vi "REMOND Studio_EC Water Q.vi"() -> ()   [LabVIEW 2021]
uses:
  FSM_States.ctl
  Global_Message.ctl
  <vilib>/Utility/error.llb/DialogType.ctl
  <vilib>/Modbus/master/Modbus Master.lvclass
  Global_flags.vi
  <vilib>/Modbus/master/Create Master Instance (Serial).vi
panel:
  in  "D.S":u16(ring)=1 items=["0.5s", "1s", "1.5s", "2.0s", "2.5s", "3.0s", "3.5s", "4.0s", "4.5s", "5.0s"]
  out "New EC":sgl=1.0
  in  "Standard Sol [mS/cm].":sgl=1.413
  in  "Set K=1":bool
  in  "Confirm EC":bool
  in  "BaudRate (9600)":u32=9600
  in  "Address":u8=1
  in  "Open/Close COM":bool
  in  "COM":refnum<visa-resource-name>
  out "Salinity:":sgl
  out "TDS:":sgl
  out "Temperature [°C]:":sgl
  out "Resistivity [ohm.cm]:":sgl
  in  "Exit":bool
  in  "Restore Default":bool
  out "Conductivity [mS/cm]:":sgl
  in  "Adquire / Stop":bool
  out "Consumer Shutdown":bool
  in  "SetBaudRate":bool
  in  "BaudRate (9600)":u16(ring)=2 items=["2400", "4800", "9600", "19200", "38400"]
  in  "Addr Set":u16=1
  in  "SetAddress":bool
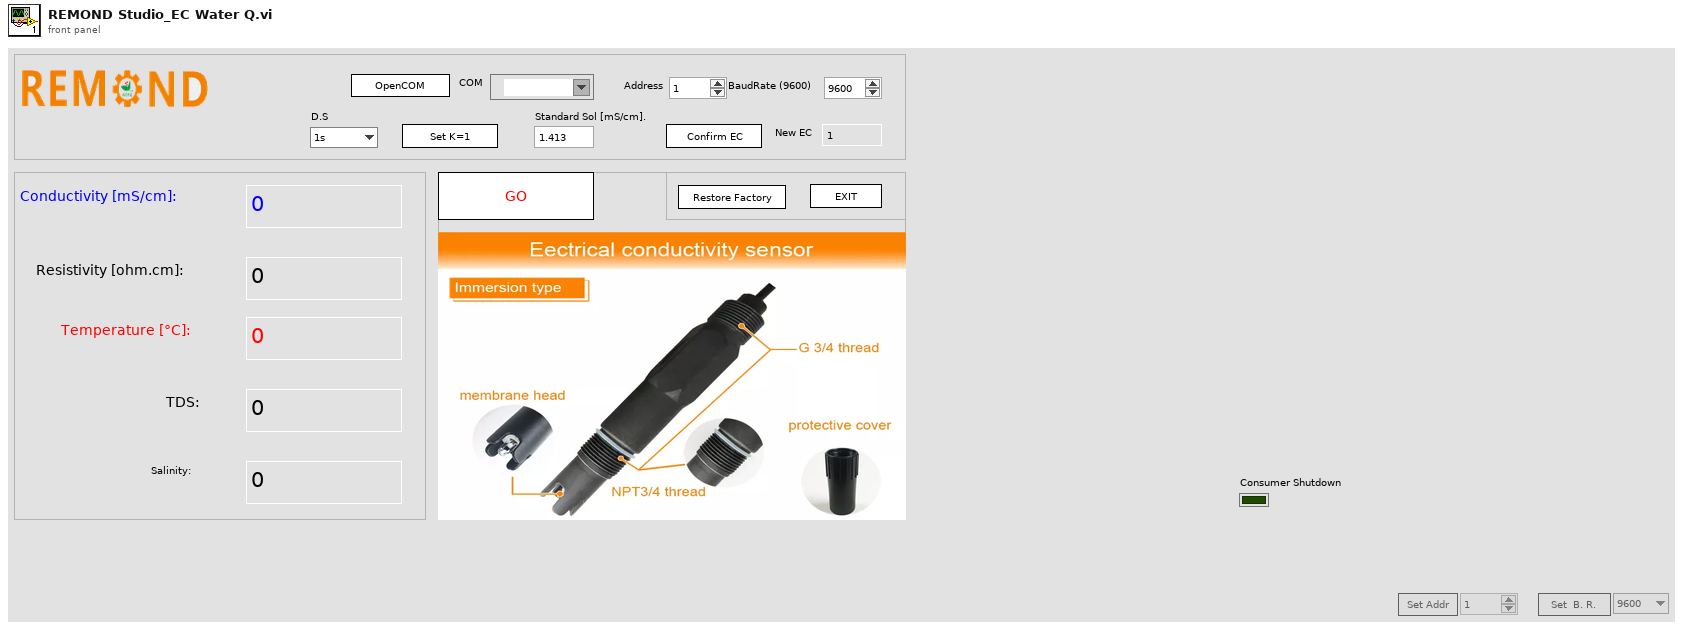
[diagram p1: front panel]
types:
  T1 = typedef "Global_Message.ctl" = cluster{"Consumer State":T2, "User Msg":string, "error in (no error)":errorcluster, "User Msg 2":string}
  T2 = typedef "FSM_States.ctl" = enum16{"Initialize", "Open COM Port", "Adquire Data", "Set Address", "Set BaudRate", "Restore Factory", "Pre-Set Zero", "Pre-Set K=1", "Pre-Set Slope", "Confirm Zero", "Confirm Slope", "Confirm EC", "Close COM Port", "Exit App", "Stop Data", "Calibrate sensor"}
  T3 = typedef "DialogType.ctl" = u16
  T4 = enum8{"Enabled", "Disabled", "Disabled and Grayed Out"}
  T5 = cluster{"Conductivity":sgl, "Resistivity":sgl, "Temperature":sgl, "TDS":sgl, "Salinity":sgl}
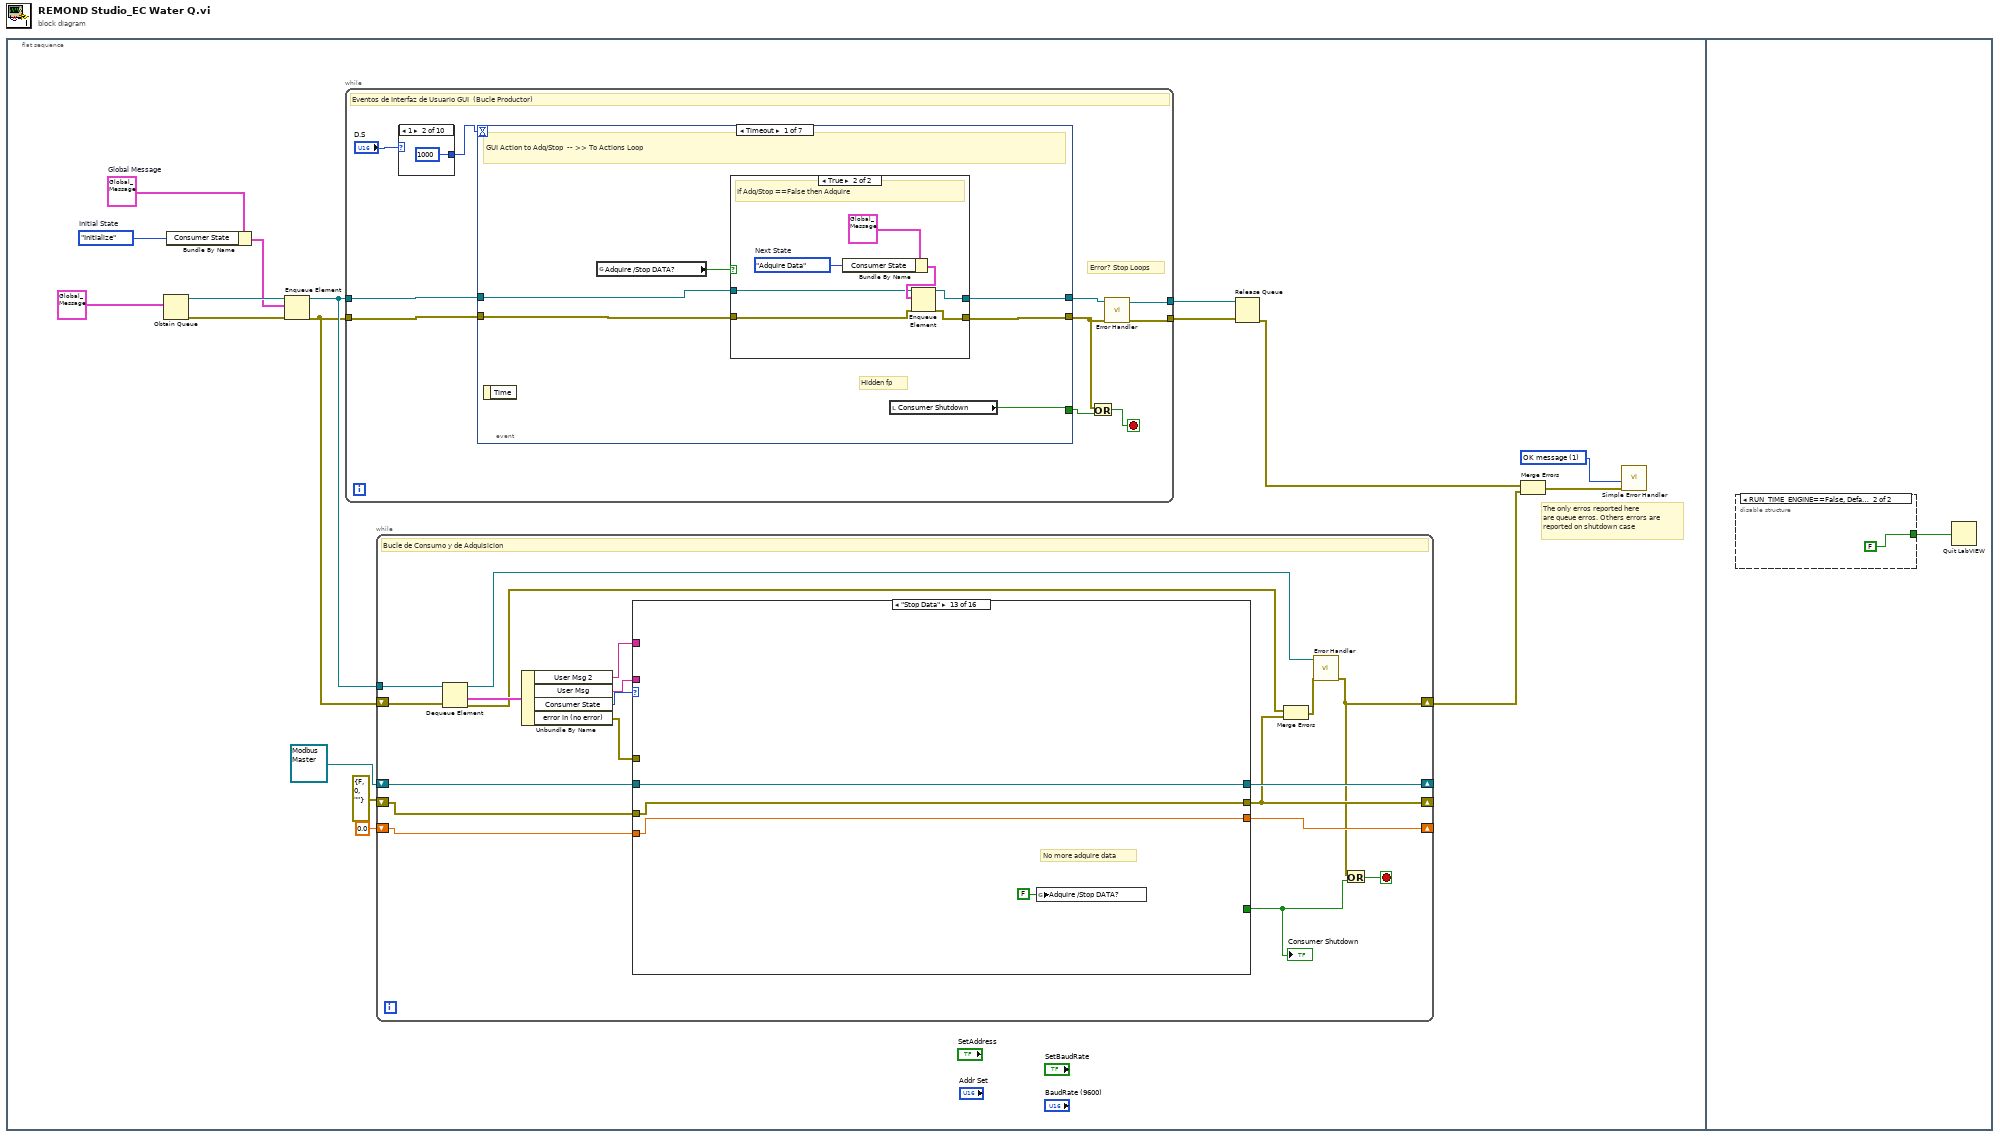
[diagram p0: block diagram]
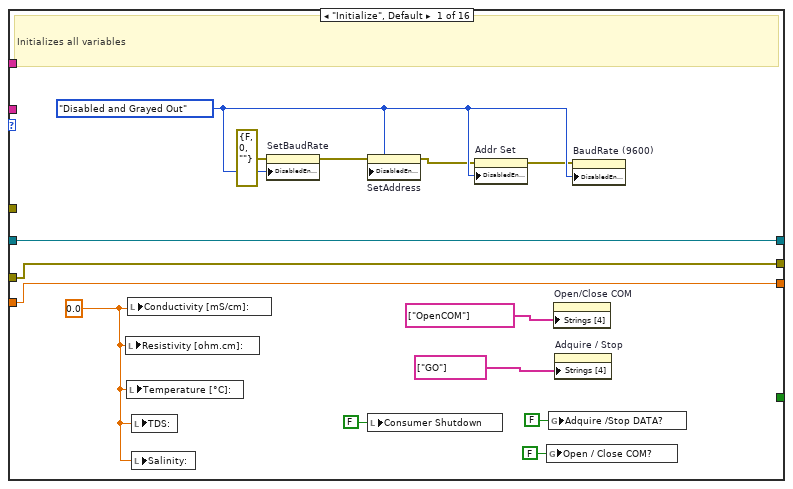
[diagram p2: hidden frame]
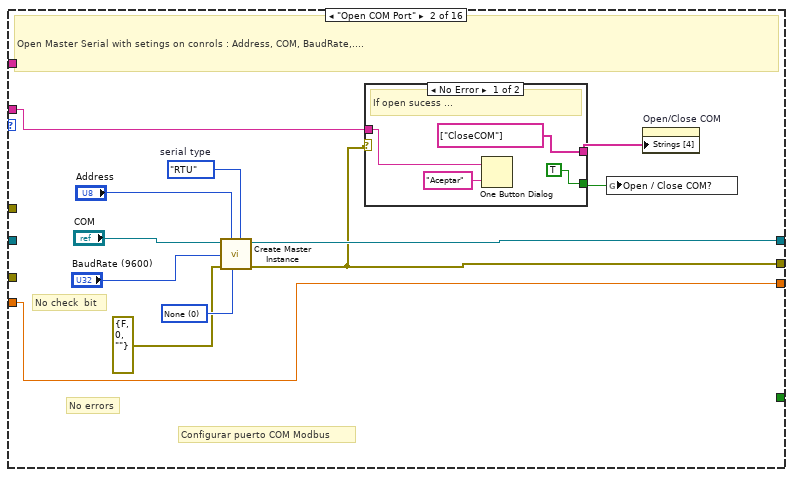
[diagram p3: hidden frame]
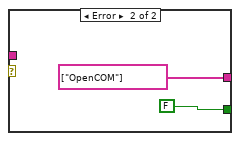
[diagram p4: hidden frame]
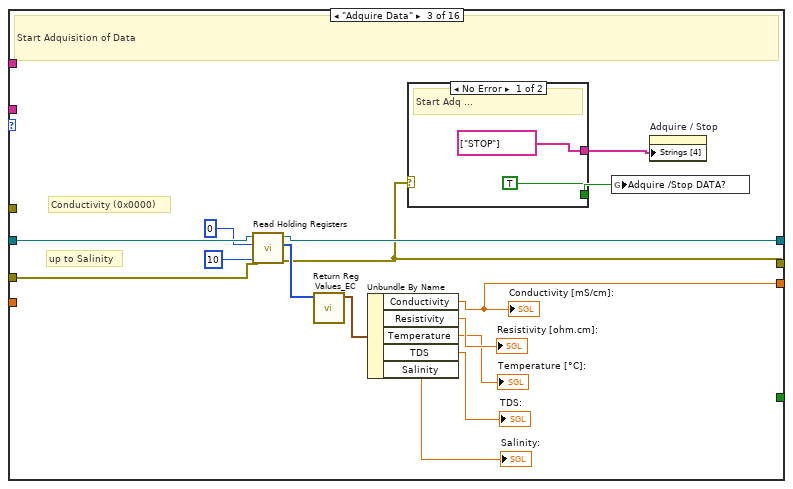
[diagram p5: hidden frame]
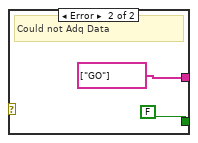
[diagram p6: hidden frame]
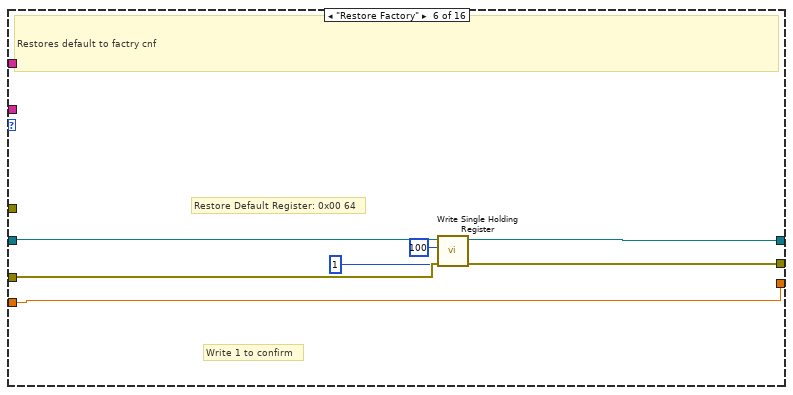
[diagram p9: hidden frame]
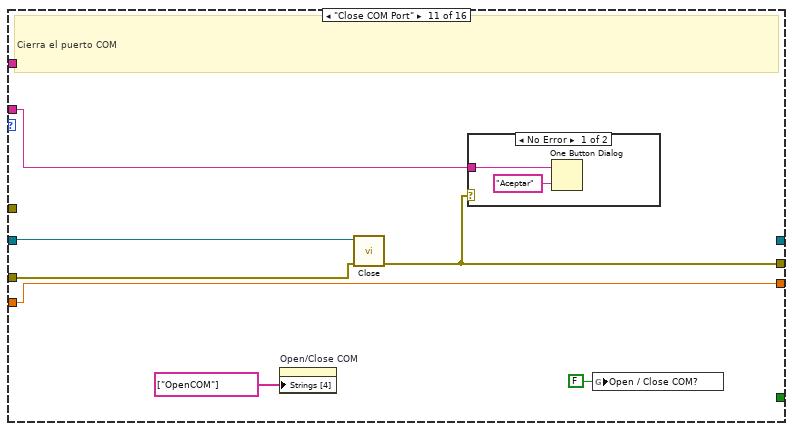
[diagram p14: hidden frame]
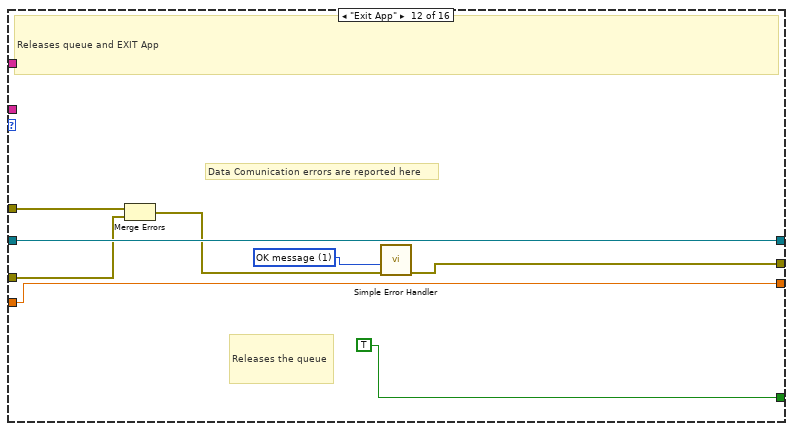
[diagram p16: hidden frame]
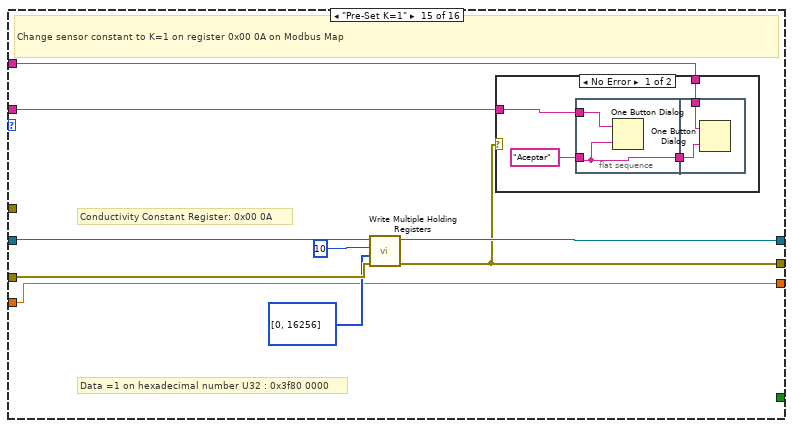
[diagram p18: hidden frame]
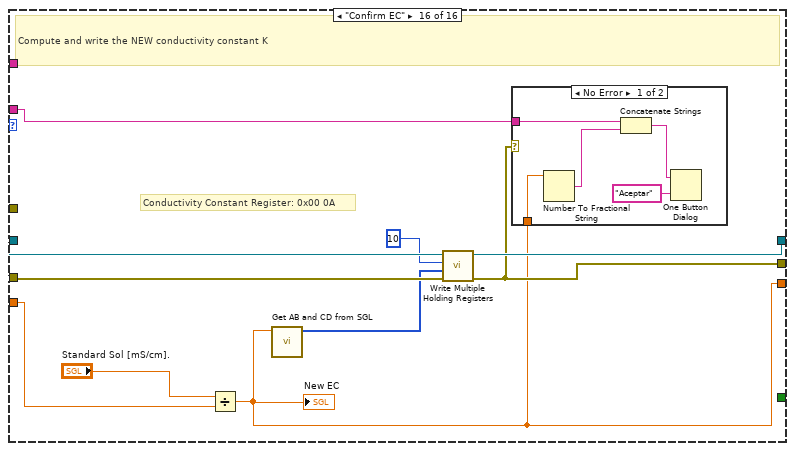
[diagram p20: hidden frame]
diagram:
  n1 = flat-sequence {
    frame #0 {
      w3 = T3 1 items=["no dialog", "OK message", "continue or stop message", "OK message + warnings", "continue/stop + warnings"] ("type of dialog (OK msg:1)")
      w14 = T1 {"Consumer State"=enum."Open COM Port", "User Msg"="", "error in (no error)"={"status"=FALSE, "code"=0, "source"=""}, "User Msg 2"=""}  # Global Message
      w13 = FSM_States."Initialize"  # Initial State
      # "The only erros reported here\nare queue erros. Others errors are\nreported on shutdown case"
      n2 = Obtain Queue(element data type=T1 {"Consumer State"=enum."Open COM Port", "User Msg"="", "error in (no error)"={"status"=FALSE, "code"=0, "source"=""}, "User Msg 2"=""} ("Global Message")) -> (queue out=w16:refnum<queue>, error out=w15:errorcluster)  [unwired: 4 in, 1 out]
      n3 = Bundle By Name(cluster=w14, "Consumer State"=w13) -> (w12:T1)
      n4 = Enqueue Element(queue=w16, element=w12, error in (no error)=w15) -> (queue out=w9:refnum<queue>, error out=w8:errorcluster)  [unwired: 1 in, 1 out]
      n5 = while {
        tunnel: w9 -> [w178]
        tunnel: w8 -> [w177]
        tunnel: [w175] -> w11
        tunnel: [w174] -> w10
        stop <- w173 stop-if-true
        # "Error? Stop Loops"
        # "Eventos de Interfaz de Usuario GUI  (Bucle Productor)"
        n6 = case shown="1" "D.S" {
          tunnel: [500 1000 1500 2000 2500 3000 3500 4000 4500 5000] -> w170
          frame 0, Default {
          }
          frame 1 {
          }
          frame 2 {
          }
          frame 3 {
          }
          frame 4 {
          }
          frame 5 {
          }
          frame 6 {
          }
          frame 7 {
          }
          frame 8 {
          }
          frame 9 {
          }
        }
        n7 = event shown="[0] Timeout" {
          selector: _ -> [_ _ _ _ _ _ _]
          dyn-events: _ -> [_ _ _ _ _ _ _]
          timeout: w170 -> [_ _ _ _ _ _ _]
          tunnel: w178 -> [w194 w208 w221 w242 w249 w256 w265]
          tunnel: w177 -> [w192 w207 w219 w240 w247 w254 w263]
          tunnel: [w193 w205 w220 w241 w248 w255 w264] -> w176
          tunnel: [w191 w204 w218 w239 w246 w253 w262] -> w172
          tunnel: [w189 _ _ _ _ _ TRUE] -> w169
          event Timeout {
            # "Hidden fp"
            # "GUI Action to Adq/Stop  -- >> To Actions Loop"
            n8 = event-data() -> ()  [unwired: 1 in, 1 out]
            n9 = global read "Global_flags.vi" "Adquire /Stop DATA?"() -> (w190:bool)
            n10 = case shown="True" w190 {
              tunnel: w194 -> [w196 w201]
              tunnel: [w196 w200] -> w193
              tunnel: w192 -> [w195 w199]
              tunnel: [w195 w198] -> w191
              frame False {
                # "Otherwise bypass..."
              }
              frame True {
                w197 = FSM_States."Adquire Data"  # Next State
                # "If Adq/Stop ==False then Adquire"
                n11 = Bundle By Name(cluster=T1 {"Consumer State"=enum."Open COM Port", "User Msg"="", "error in (no error)"={"status"=FALSE, "code"=0, "source"=""}, "User Msg 2"=""} ("Global Message"), "Consumer State"=w197) -> (w202:T1)
                n12 = Enqueue Element(queue=w201, element=w202, error in (no error)=w199) -> (queue out=w200:refnum<queue>, error out=w198:errorcluster)  [unwired: 1 in, 1 out]
              }
            }
            n13 = local read "Consumer Shutdown"() -> (w189:bool)
          }
          event "Open/Close COM": Value Change {
            w213 = FSM_States."Close COM Port"  # Next State
            w214 = FSM_States."Open COM Port"  # Next State
            # "GUI Action to Open COM Port  -- >> To Actions Loop"
            n14 = event-data() -> ()  [unwired: 1 in, 1 out]
            n15 = global read "Global_flags.vi" "Open / Close COM?"() -> (w210:bool)
            n16 = Select(t="COM cerrado !", s=w210, f="Puerto COM abierto !" ("User Msg")) -> (s? t:f=w209:string)
            n17 = Select(t=w213, s=w210, f=w214) -> (s? t:f=w216:T2)
            n18 = Bundle By Name(cluster=T1 {"Consumer State"=enum."Open COM Port", "User Msg"="", "error in (no error)"={"status"=FALSE, "code"=0, "source"=""}, "User Msg 2"=""} ("Global Message"), "Consumer State"=w216, "User Msg"=w209) -> (w206:T1)
            n19 = Enqueue Element(queue=w208, element=w206, error in (no error)=w207) -> (queue out=w205:refnum<queue>, error out=w204:errorcluster)  [unwired: 1 in, 1 out]
          }
          event "Adquire / Stop": Value Change {
            # "! Adq has started ?"
            # "GUI Action to Adquire / Stop  -- >> To Actions Loop"
            n20 = event-data() -> ()  [unwired: 1 in, 1 out]
            n21 = global read "Global_flags.vi" "Adquire /Stop DATA?"() -> (w217:bool)
            n22 = case shown="True" w217 {
              tunnel: w221 -> [w226 w232]
              tunnel: [w225 w231] -> w220
              tunnel: w219 -> [w224 w229]
              tunnel: [w223 w230] -> w218
              frame False {
                w222 = FSM_States."Adquire Data"  # Next State
                # "If no Adq started, then Start adquiring .."
                n23 = Bundle By Name(cluster=T1 {"Consumer State"=enum."Open COM Port", "User Msg"="", "error in (no error)"={"status"=FALSE, "code"=0, "source"=""}, "User Msg 2"=""} ("Global Message"), "Consumer State"=w222) -> (w227:T1)
                n24 = Enqueue Element(queue=w226, element=w227, error in (no error)=w224) -> (queue out=w225:refnum<queue>, error out=w223:errorcluster)  [unwired: 1 in, 1 out]
              }
              frame True {
                w233 = FSM_States."Stop Data"  # Next State
                # "Otherwise STOP Adq"
                n25 = Bundle By Name(cluster=T1 {"Consumer State"=enum."Open COM Port", "User Msg"="", "error in (no error)"={"status"=FALSE, "code"=0, "source"=""}, "User Msg 2"=""} ("Global Message"), "Consumer State"=w233) -> (w234:T1)
                n26 = Enqueue Element(queue=w232, element=w234, error in (no error)=w229) -> (queue out=w231:refnum<queue>, error out=w230:errorcluster)  [unwired: 1 in, 1 out]
              }
            }
          }
          event "Set K=1": Value Change {
            w243 = FSM_States."Pre-Set K=1"  # Next State
            # "GUI Action to \"Set K=1\"  -- >> To Actions Loop"
            n27 = event-data() -> ()  [unwired: 1 in, 1 out]
            n28 = Bundle By Name(cluster=T1 {"Consumer State"=enum."Open COM Port", "User Msg"="", "error in (no error)"={"status"=FALSE, "code"=0, "source"=""}, "User Msg 2"=""} ("Global Message"), "Consumer State"=w243, "User Msg"="OK Set K=1 !! ", "User Msg 2"="Colocar sensor en Liqu de calibracion. " ("User Msg")) -> (w238:T1)
            n29 = Enqueue Element(queue=w242, element=w238, error in (no error)=w240) -> (queue out=w241:refnum<queue>, error out=w239:errorcluster)  [unwired: 1 in, 1 out]
          }
          event "Confirm EC": Value Change {
            w252 = FSM_States."Confirm EC"  # Next State
            # "GUI Action to Confirm EC  -- >> To Actions Loop"
            n30 = event-data() -> ()  [unwired: 1 in, 1 out]
            n31 = Bundle By Name(cluster=T1 {"Consumer State"=enum."Open COM Port", "User Msg"="", "error in (no error)"={"status"=FALSE, "code"=0, "source"=""}, "User Msg 2"=""} ("Global Message"), "Consumer State"=w252, "User Msg"="OK Set K=") -> (w250:T1)
            n32 = Enqueue Element(queue=w249, element=w250, error in (no error)=w247) -> (queue out=w248:refnum<queue>, error out=w246:errorcluster)  [unwired: 1 in, 1 out]
          }
          event "Restore Default": Value Change {
            w260 = FSM_States."Restore Factory"  # Next State
            # "GUI Action to Restore Default  -- >> To Actions Loop"
            n33 = event-data() -> ()  [unwired: 1 in, 1 out]
            n34 = Bundle By Name(cluster=T1 {"Consumer State"=enum."Open COM Port", "User Msg"="", "error in (no error)"={"status"=FALSE, "code"=0, "source"=""}, "User Msg 2"=""} ("Global Message"), "Consumer State"=w260, "User Msg"="OK Restore Fact !") -> (w258:T1)
            n35 = Enqueue Element(queue=w256, element=w258, error in (no error)=w254) -> (queue out=w255:refnum<queue>, error out=w253:errorcluster)  [unwired: 1 in, 1 out]
          }
          event "Exit": Value Change {
            w267 = FSM_States."Exit App"  # Next State
            n36 = event-data() -> ()  [unwired: 1 in, 1 out]
            n37 = Bundle By Name(cluster=T1 {"Consumer State"=enum."Open COM Port", "User Msg"="", "error in (no error)"={"status"=FALSE, "code"=0, "source"=""}, "User Msg 2"=""} ("Global Message"), "Consumer State"=w267) -> (w266:T1)
            n38 = Enqueue Element At Opposite End(queue=w265, element=w266, error in (no error)=w263) -> (queue out=w264:refnum<queue>, error out=w262:errorcluster)  [unwired: 1 in, 1 out]
          }
        }
        n39 = Or(x=w172, y=w169) -> (x .or. y?=w173:bool)
        n40 = call "Error Handler.vi"("error in (no error)"=w172, "Queue in"=w176) -> ("error out"=w174:errorcluster, "Queue out"=w175:refnum<queue>)  [unwired: 8 in]
      }
      n41 = while {
        tunnel: w9 -> [w36]
        shift-right: [w32] -> _
        shift-left: refnum<class "Modbus Master.lvclass"> refnum ("Modbus master out") -> [w30]
        shift-right: [w28] -> _
        shift-left: errorcluster {"status"=FALSE, "code"=0, "source"=""} ("error out") -> [w29]
        shift-right: [w24] -> _
        shift-left: sgl 0.0 ("Conductivity") -> [w23]
        shift-right: [w19] -> w5
        shift-left: w8 -> [w35]
        stop <- w22 stop-if-true
        # "Bucle de Consumo y de Adquisicion"
        n42 = Dequeue Element(queue=w36, error in (no error)=w35) -> (queue out=w27:refnum<queue>, element=w34:T1, error out=w26:errorcluster)  [unwired: 1 in, 1 out]
        n43 = Unbundle By Name(w34) -> ("User Msg 2"=w25:string, "User Msg"=w31:string, "Consumer State"=w33:T2, "error in (no error)"=w18:errorcluster)
        n44 = case shown="\"Stop Data\"" w33 {
          tunnel: [w46 w56 w82 w90 w93 w99 w103 w106 w109 w112 _ w129 w133 w136 w144 w160] -> w32
          tunnel: [w37 w55 w72 w89 w92 w97 w102 w105 w108 w111 w116 w126 w132 w135 w140 w156] -> w28
          tunnel: w31 -> [_ w53 _ _ _ _ _ _ _ _ w115 _ _ _ w139 w154]
          tunnel: w30 -> [w46 _ w83 w90 w93 w100 w103 w106 w109 w112 w117 w129 w133 w136 w145 w161]
          tunnel: w29 -> [w37 _ w79 w89 w92 w98 w102 w105 w108 w111 w118 w123 w132 w135 w143 w159]
          tunnel: w25 -> [_ _ _ _ _ _ _ _ _ _ _ _ _ _ w138 _]
          tunnel: [w45 w51 w69 w88 w91 w94 w101 w104 w107 w110 w119 w128 w131 w134 w137 w155] -> w24
          tunnel: w23 -> [w45 w51 _ w88 w91 w94 w101 w104 w107 w110 w119 w128 w131 w134 w137 w162]
          tunnel: [_ _ _ _ _ _ _ _ _ _ _ TRUE _ _ _ _] -> w21
          tunnel: w18 -> [_ _ _ _ _ _ _ _ _ _ _ w124 _ _ _ _]
          frame "Initialize", Default {
            w44 = sgl 0.0 ("Conductivity [mS/cm]:")
            w50 = T4."Disabled and Grayed Out" ("Disabled")
            # "Initializes all variables"
            n45 = local write "Resistivity [ohm.cm]:"(w44) -> ()
            n46 = local write "Temperature [°C]:"(w44) -> ()
            n47 = local write "Conductivity [mS/cm]:"(w44) -> ()
            n48 = local write "TDS:"(w44) -> ()
            n49 = local write "Salinity:"(w44) -> ()
            n50 = property on="SetBaudRate" class="Bool"(error in=errorcluster {"status"=FALSE, "code"=0, "source"=""} ("error in (no error)"), "DisabledEnum"=w50) -> (error out=w49:errorcluster)  [unwired: 1 in, 1 out]
            n51 = property on="SetAddress" class="Bool"(error in=w49, "DisabledEnum"=w50) -> (error out=w48:errorcluster)  [unwired: 1 in, 1 out]
            n52 = local write "Consumer Shutdown"(FALSE ("Consumer Shutdown")) -> ()
            n53 = property on="Addr Set" class="DigNum (strict)"(error in=w48, "DisabledEnum"=w50) -> (error out=w47:errorcluster)  [unwired: 1 in, 1 out]
            n54 = global write "Global_flags.vi" "Open / Close COM?"(FALSE ("Open / Close COM?")) -> ()
            n55 = global write "Global_flags.vi" "Adquire /Stop DATA?"(FALSE ("Adquire /Stop DATA?")) -> ()
            n56 = property on="Open/Close COM" class="Bool"("Strings [4]"=string[] ["OpenCOM"]) -> ()  [unwired: 2 in, 2 out]
            n57 = property on="Adquire / Stop" class="Bool"("Strings [4]"=string[] ["GO"]) -> ()  [unwired: 2 in, 2 out]
            n58 = property on="BaudRate (9600)" class="Ring (strict)"(error in=w47, "DisabledEnum"=w50) -> ()  [unwired: 1 in, 2 out]
          }
          frame "Open COM Port" {
            w58 = u16 0 items=["None", "Odd", "Even"] ("parity (Even)")
            w60 = enum16{"RTU", "ASCII"}."RTU"  # serial type
            # "No errors"
            # "No check  bit"
            # "Configurar puerto COM Modbus"
            # "Open Master Serial with setings on conrols : Address, COM, BaudRate,...."
            n59 = call-poly <vilib>:"Create Master Instance.vi"("serial type"=w60, "parity (Even)"=w58, "unit ID"="Address", "error in (no error)"=errorcluster {"status"=FALSE, "code"=0, "source"=""}, "baud rate (9600)"="BaudRate (9600)", "VISA resource name"="COM") -> ("error out"=w55:errorcluster, "serial master instance"=w56:refnum<class "Modbus Master.lvclass">)  [unwired: 4 in]
            n60 = case shown="No Error" w55 {
              tunnel: [string[] ["CloseCOM"] ("Strings [4]") string[] ["OpenCOM"] ("Strings [4]")] -> w54
              tunnel: w53 -> [w65 _]
              tunnel: [TRUE ("Open / Close COM?") FALSE ("Open / Close COM?")] -> w52
              frame No Error {
                # "If open sucess ..."
                n61 = One Button Dialog(message=w65, button name ("OK")="Aceptar") -> ()  [unwired: 1 out]
              }
              frame Error {
              }
            }
            n62 = global write "Global_flags.vi" "Open / Close COM?"(w52) -> ()
            n63 = property on="Open/Close COM" class="Bool"("Strings [4]"=w54) -> ()  [unwired: 2 in, 2 out]
          }
          frame "Adquire Data" {
            # "up to Salinity"
            # "Conductivity (0x0000)"
            # "Start Adquisition of Data"
            n64 = call-dynamic "Read Holding Registers.vi"("error in (no error)"=w79, "number of holding registers"=u16 10, "starting address"=u16 0, "Modbus master in"=w83) -> ("error out"=w72:errorcluster, "register values"=w78:u16[], "Modbus master out"=w82:refnum<class "Modbus Master.lvclass">)  [unwired: 5 in]
            n65 = call "Return Reg Values_EC.vi"("Modbus Register Map"=w78) -> ("EC Values"=w77:T5)  [unwired: 10 in]
            n66 = Unbundle By Name(w77) -> ("Conductivity"=w69:sgl, "Resistivity"=→"Resistivity [ohm.cm]:":sgl, "Temperature"=→"Temperature [°C]:":sgl, "TDS"=→"TDS:":sgl, "Salinity"=→"Salinity:":sgl)
            "Conductivity [mS/cm]:" <- w69
            n67 = case shown="No Error" w72 {
              tunnel: [TRUE FALSE] -> w71
              tunnel: [string[] ["STOP"] ("Strings [4]") string[] ["GO"] ("Strings [4]")] -> w70
              frame No Error {
                # "Start Adq ..."
              }
              frame Error {
                # "Could not Adq Data"
              }
            }
            n68 = global write "Global_flags.vi" "Adquire /Stop DATA?"(w71) -> ()
            n69 = property on="Adquire / Stop" class="Bool"("Strings [4]"=w70) -> ()  [unwired: 2 in, 2 out]
          }
          frame "Set Address" {
          }
          frame "Set BaudRate" {
          }
          frame "Restore Factory" {
            # "Write 1 to confirm"
            # "Restore Default Register: 0x00 64"
            # "Restores default to factry cnf"
            n70 = call-dynamic "Write Single Holding Register.vi"("error in (no error)"=w98, "holding register value"=u16 1, "address"=u16 100, "Modbus master in"=w100) -> ("error out"=w97:errorcluster, "Modbus master out"=w99:refnum<class "Modbus Master.lvclass">)  [unwired: 6 in]
          }
          frame "Pre-Set Zero" {
          }
          frame "Pre-Set Slope" {
          }
          frame "Confirm Zero" {
          }
          frame "Confirm Slope" {
          }
          frame "Close COM Port" {
            # "Cierra el puerto COM"
            n71 = property on="Open/Close COM" class="Bool"("Strings [4]"=string[] ["OpenCOM"]) -> ()  [unwired: 2 in, 2 out]
            n72 = call-dynamic "Close.vi"("error in (no error)"=w118, "Modbus master in"=w117) -> ("error out"=w116:errorcluster)  [unwired: 9 in]
            n73 = case shown="No Error" w116 {
              tunnel: w115 -> [w121 _]
              frame No Error {
                n74 = One Button Dialog(message=w121, button name ("OK")="Aceptar") -> ()  [unwired: 1 out]
              }
              frame Error {
              }
            }
            n75 = global write "Global_flags.vi" "Open / Close COM?"(FALSE ("Open / Close COM?")) -> ()
          }
          frame "Exit App" {
            w125 = T3 1 items=["no dialog", "OK message", "continue or stop message", "OK message + warnings", "continue/stop + warnings"] ("type of dialog (OK msg:1)")
            # "Data Comunication errors are reported here"
            # "Releases the queue"
            # "Releases queue and EXIT App"
            n76 = Merge Errors(w124, w123) -> (w122:errorcluster)
            n77 = call <vilib>:"Simple Error Handler.vi"("type of dialog (OK msg:1)"=w125, "error in (no error)"=w122) -> ("error out"=w126:errorcluster)  [unwired: 3 in, 4 out]
          }
          frame "Stop Data" {
            # "No more adquire data"
            n78 = global write "Global_flags.vi" "Adquire /Stop DATA?"(FALSE ("Adquire /Stop DATA?")) -> ()
          }
          frame "Calibrate sensor" {
          }
          frame "Pre-Set K=1" {
            # "Data =1 on hexadecimal number U32 : 0x3f80 0000"
            # "Conductivity Constant Register: 0x00 0A"
            # "Change sensor constant to K=1 on register 0x00 0A on Modbus Map"
            n79 = call-dynamic "Write Multiple Holding Registers.vi"("error in (no error)"=w143, "holding register values"=u16[] [0, 16256], "starting address"=u16 10, "Modbus master in"=w145) -> ("error out"=w140:errorcluster, "Modbus master out"=w144:refnum<class "Modbus Master.lvclass">)  [unwired: 6 in]
            n80 = case shown="No Error" w140 {
              tunnel: w139 -> [w149 _]
              tunnel: w138 -> [w146 _]
              frame No Error {
                n81 = flat-sequence {
                  tunnel: w149 -> [w151]
                  tunnel: "Aceptar" ("button name (\"OK\")") -> [w150]
                  tunnel: [w150] -> w147
                  tunnel: w147 -> [w153]
                  tunnel: w146 -> [w152]
                  frame #0 {
                    n82 = One Button Dialog(message=w151, button name ("OK")=w150) -> ()  [unwired: 1 out]
                  }
                  frame #1 {
                    n83 = One Button Dialog(message=w152, button name ("OK")=w153) -> ()  [unwired: 1 out]
                  }
                }
              }
              frame Error {
              }
            }
          }
          frame "Confirm EC" {
            # "Conductivity Constant Register: 0x00 0A"
            # "Compute and write the NEW conductivity constant K"
            n84 = Divide(x="Standard Sol [mS/cm].", y=w162) -> (x/y=w155:sgl)
            "New EC" <- w155
            n85 = call "Get AB and CD from SGL.vi"("Float Number In"=w155) -> ("CD\nAB"=w157:u16[])  [unwired: 10 in]
            n86 = call-dynamic "Write Multiple Holding Registers.vi"("error in (no error)"=w159, "holding register values"=w157, "starting address"=u16 10, "Modbus master in"=w161) -> ("error out"=w156:errorcluster, "Modbus master out"=w160:refnum<class "Modbus Master.lvclass">)  [unwired: 6 in]
            n87 = case shown="No Error" w156 {
              tunnel: w155 -> [w168 _]
              tunnel: w154 -> [w167 _]
              frame No Error {
                n88 = Number To Fractional String(number=w168) -> (F-format string=w164:string)  [unwired: 3 in]
                n89 = Concatenate Strings(w167, w164) -> (w166:string)
                n90 = One Button Dialog(message=w166, button name ("OK")="Aceptar") -> ()  [unwired: 1 out]
              }
              frame Error {
              }
            }
          }
        }
        "Consumer Shutdown" <- w21
        n91 = Merge Errors(w26, w28) -> (w20:errorcluster)
        n92 = call "Error Handler.vi"("error in (no error)"=w20, "Queue in"=w27) -> ("error out"=w19:errorcluster)  [unwired: 8 in, 1 out]
        n93 = Or(x=w19, y=w21) -> (x .or. y?=w22:bool)
      }
      n94 = Release Queue(queue=w11, error in (no error)=w10) -> (error out=w6:errorcluster)  [unwired: 1 in, 2 out]
      n95 = Merge Errors(w6, w5) -> (w4:errorcluster)
      n96 = call <vilib>:"Simple Error Handler.vi"("type of dialog (OK msg:1)"=w3, "error in (no error)"=w4) -> ()  [unwired: 3 in, 5 out]
    }
    frame #1 {
      n97 = disable-structure shown="RUN_TIME_ENGINE==False, Default" {
        disable-tunnel: [TRUE FALSE] -> w269
        frame condition #0 {
        }
        frame condition #1 (active) {
        }
      }
      n98 = Quit LabVIEW(quit? (T)=w269) -> ()
    }
  }
